vi "LoggingData.vi"(8 "error in (no error)":errorcluster, 10 "Start time":u32, 11 "Refmum":refnum<file>) -> (0 "error out":errorcluster, 3 "Byte Stream File out":refnum<file>)   [LabVIEW 2017]
uses:
  DataNames.ctl
  LogOperation.ctl
  Framework/Robot Global Data.vi
  <vilib>/NI_Real-Time Target Support.lvlib
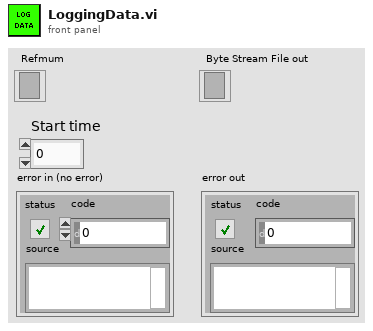
[diagram p1: front panel]
types:
  T1 = typedef "DataNames.ctl" = enum16{"RobotMode", "FMSConnected", "DriveLeft", "DriveRight", "EncoderLeft", "EncoderRight", "Angle", "LocationX", "LocationY", "CPU1", "CPU2", "DriveOperation", "Battery"}
  T2 = typedef "LogOperation.ctl" = enum16{"Set", "Get All", "Init"}
  T3 = typedef "NI_Real-Time Target Support.lvlib/RT CPU Load.ctl" = cluster{"Total (%)":dbl, "Time Critical (%)":dbl, "Timed Structures (%)":dbl, "High (%)":dbl, "Above Normal (%)":dbl, "Normal (%)":dbl, "Background (%)":dbl, "Idle (%)":dbl, "ISR (%)":dbl}
  T4 = typedef "WPI_DriverStationRobotMode2.ctl" = enum16{"Autonomous Disabled", "Autonomous Enabled", "Teleop Disabled", "Teleop Enabled", "Disconnected", "Finish", "Test Disabled", "Test Enabled", "Emergency Stopped"}
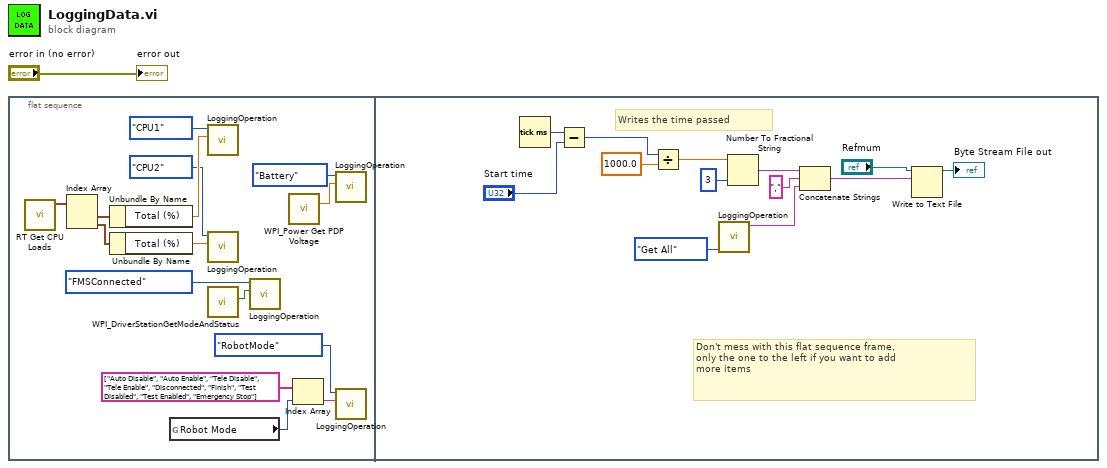
[diagram p0: block diagram]
diagram:
  n1 = flat-sequence {
    frame #0 {
      n2 = call <vilib>:"RT Get CPU Loads.vi"() -> ("CPU loads"=w12:T3[])  [unwired: 10 in, 1 out]
      n3 = Index Array(array=w12) -> (element #1=w13:T3, element #2=w14:T3)  [unwired: 2 in]
      n4 = Unbundle By Name(w13) -> ("Total (%)"=w15:dbl)
      n5 = Unbundle By Name(w14) -> ("Total (%)"=w16:dbl)
      n6 = global read "Robot Global Data.vi" "Robot Mode"() -> (w9:T4)
      n7 = call "LoggingOperation.vi"("Data"=w15, "Name"=DataNames."CPU1") -> ()  [unwired: 9 in, 1 out]
      n8 = call "LoggingOperation.vi"("Data"=w16, "Name"=DataNames."CPU2") -> ()  [unwired: 9 in, 1 out]
      n9 = call <vilib>:"WPI_DriverStationGetModeAndStatus.vi"() -> ("FMS Attached"=w10:bool)  [unwired: 10 in, 1 out]
      n10 = call "LoggingOperation.vi"("Data"=w10, "Name"=DataNames."FMSConnected") -> ()  [unwired: 9 in, 1 out]
      n11 = call <vilib>:"WPI_Power Get PDP Voltage.vi"() -> ("voltage (V)"=w2:dbl)  [unwired: 14 in, 1 out]
      n12 = Index Array(array=string[] ["Auto Disable", "Auto Enable", "Tele Disable", "Tele Enable", "Disconnected", "Finish", "Test Disabled", "Test Enabled", "Emergency Stop"], index=w9) -> (element=w11:string)
      n13 = call "LoggingOperation.vi"("Data"=w2, "Name"=DataNames."Battery") -> ()  [unwired: 9 in, 1 out]
      n14 = call "LoggingOperation.vi"("Data"=w11, "Name"=DataNames."RobotMode") -> ()  [unwired: 9 in, 1 out]
    }
    frame #1 {
      # "Don't mess with this flat sequence frame,\nonly the one to the left if you want to add\nmore items"
      # "Writes the time passed"
      n15 = Tick Count (ms)() -> (millisecond timer value=w29:u32)
      n16 = Subtract(x=w29, y="Start time") -> (x-y=w27:u32)
      n17 = Divide(x=w27, y=1000.0 ("input 9")) -> (x/y=w22:dbl)
      n18 = call "LoggingOperation.vi"("Operation"=LogOperation."Get All") -> ("Log String"=w18:string)  [unwired: 10 in]
      n19 = Number To Fractional String(number=w22, precision (6)=i16 3) -> (F-format string=w20:string)  [unwired: 2 in]
      n20 = Concatenate Strings(w20, "," ("string"), w18) -> (w17:string)
      n21 = Write to Text File(file (use dialog)="Refmum", text=w17) -> (refnum out=→"Byte Stream File out":refnum<file>)  [unwired: 2 in, 2 out]
    }
  }
  "error out" <- "error in (no error)"
